vi "GET_Snapshotdata_by_id.vi"(8 "SnapID":string, 11 "API Key":string="cheia04042025tema2restfulapi") -> (2 "headers":string, 3 "Diagnose snapshot":string)   [LabVIEW 2024]
uses:
  <vilib>/httpClient/LabVIEWHTTPClient.lvlib
panel:
  out "error out get":errorcluster
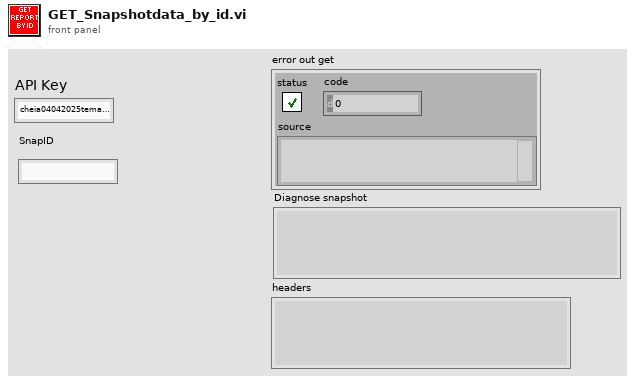
[diagram p1: front panel]
types:
  T1 = typedef "LabVIEWHTTPClient.lvlib/ClientHandle.ctl" = refnum<k1>
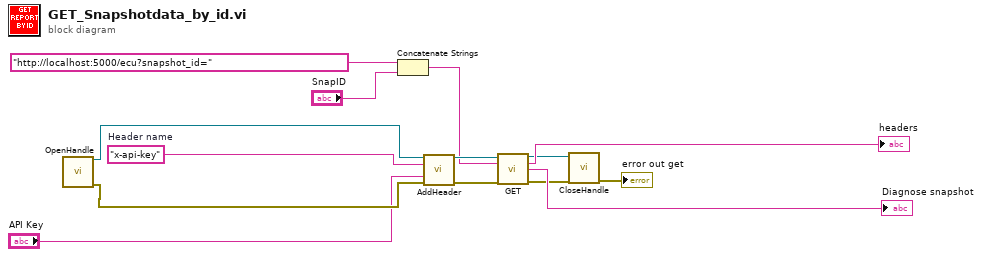
[diagram p0: block diagram]
diagram:
  w5 = "x-api-key"  # Header name
  n1 = call <vilib>:"OpenHandle.vi"() -> ("client handle out"=w6:T1, "error out"=w7:errorcluster)  [unwired: 14 in]
  n2 = Concatenate Strings("http://localhost:5000/ecu?snapshot_id=" ("url"), "SnapID") -> (w3:string)
  n3 = call <vilib>:"AddHeader.vi"("client handle"=w6, "header"=w5, "value"="API Key", "error in (no error)"=w7) -> ("client handle out"=w9:T1, "error out"=w8:errorcluster)  [unwired: 10 in]
  n4 = call <vilib>:"GET.vi"("client handle"=w9, "url"=w3, "error in (no error)"=w8) -> ("client handle out"=w11:T1, "headers"=→"headers":string, "body"=→"Diagnose snapshot":string, "error out"=w10:errorcluster)  [unwired: 9 in]
  n5 = call <vilib>:"CloseHandle.vi"("client handle"=w11, "error in (no error)"=w10) -> ("error out"=→"error out get":errorcluster)  [unwired: 13 in]
